vi "Variant_MergeElements.vi"(10 "New Element(s)":variant, 11 "Original Element(s)":variant) -> (3 "Merged Elements":variant)   [LabVIEW 2013, in "OpenVariant.lvlib"]
uses:
  OpenVariant.lvlib
  TypeDescriptor/OpenDescriptor.lvlib
  Conversions/OpenConvert.lvlib
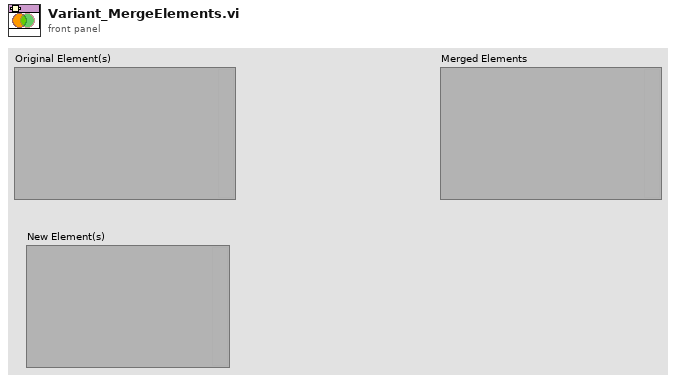
[diagram p1: front panel]
types:
  T1 = typedef "OpenDescriptor.lvlib/OpenDescriptor -- cluster.ctl" = cluster{"type descriptor":i16[], "name":string, "class":string, "data string":string}
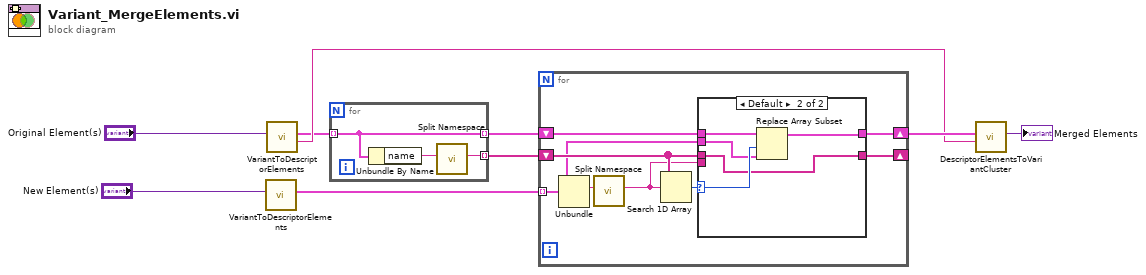
[diagram p0: block diagram]
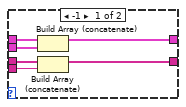
[diagram p2: hidden frame]
diagram:
  n1 = call "VariantToDescriptorElements.vi"("Variant"="New Element(s)") -> ("Descriptors"=w5:T1[])  [unwired: 9 in, 1 out]
  n2 = call "VariantToDescriptorElements.vi"("Variant"="Original Element(s)") -> ("name"=w6:string, "Descriptors"=w3:T1[])  [unwired: 9 in]
  n3 = for {
    tunnel: w3 -> [w10] mode=indexing
    tunnel: [w11] -> w9 mode=indexing
    tunnel: [w10] -> w4 mode=indexing
    n4 = Unbundle By Name(w10) -> ("name"=w12:string)
    n5 = call "Split Namespace.vi"("Namespaced String"=w12) -> ("String"=w11:string)  [unwired: 9 in, 1 out]
  }
  n6 = for {
    tunnel: w5 -> [w13] mode=indexing
    shift-right: [w19] -> w8
    shift-left: w4 -> [w20]
    shift-right: [w17] -> _
    shift-left: w9 -> [w18]
    n7 = Unbundle(w13) -> ("name"=w15:string)  [unwired: 3 out]
    n8 = call "Split Namespace.vi"("Namespaced String"=w15) -> ("String"=w14:string)  [unwired: 9 in, 1 out]
    n9 = Search 1D Array(1D array=w18, element=w14) -> (index of element=w16:i32)  [unwired: 1 in]
    n10 = case shown="Default" w16 {
      selector: w16 -> [_ w29]
      tunnel: w20 -> [w26 w30]
      tunnel: w13 -> [w25 w28]
      tunnel: [w24 w31] -> w19
      tunnel: w18 -> [w23 w27]
      tunnel: w14 -> [w22 _]
      tunnel: [w21 w27] -> w17
      frame -1 {
        n11 = Build Array (concatenate)(w26, w25) -> (w24:T1[])
        n12 = Build Array (concatenate)(w23, w22) -> (w21:string[])
      }
      frame Default {
        n13 = Replace Array Subset(array=w30, new element=w28, index=w29) -> (w31:T1[])
      }
    }
  }
  n14 = call "DescriptorElementsToVariantCluster.vi"("Cluster Name"=w6, "Descriptors"=w8) -> ("Variant Cluster"=→"Merged Elements":variant)  [unwired: 8 in]
